vi "CallingVI.vi"() -> ()   [LabVIEW 2010]
uses:
  TimerCommands.ctl
panel:
  in  "타겟 시간 (s)":dbl
  out "경과 시간":dbl
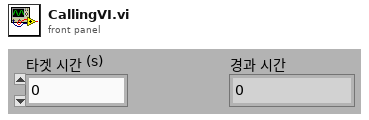
[diagram p1: front panel]
types:
  T1 = typedef "TimerCommands.ctl" = enum16{"시작", "시간 확인"}
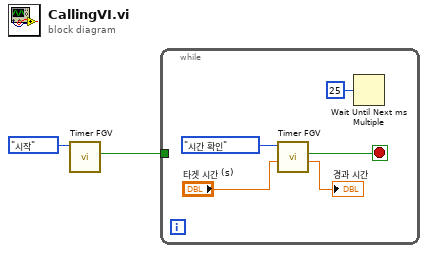
[diagram p0: block diagram]
diagram:
  n1 = call "Timer FGV.vi"("타이머 명령"=TimerCommands."시작" ("Timer Command")) -> ("완료?"=w2:bool)  [unwired: 9 in, 1 out]
  n2 = while {
    tunnel: w2 -> [_]
    stop <- w6 stop-if-true
    n3 = call "Timer FGV.vi"("타겟 시간 (s)"="타겟 시간 (s)", "타이머 명령"=TimerCommands."시간 확인" ("Timer Command")) -> ("경과 시간"=→"경과 시간":dbl, "완료?"=w6:bool)  [unwired: 8 in]
    n4 = Wait Until Next ms Multiple(millisecond multiple=u32 25) -> ()  [unwired: 1 out]
  }
